vi "Init_queue.vi"(8 "error in (no error)":errorcluster, 9 "response queue":T1, 10 "Name":string, 11 "QueueResponder in":refnum<class "QueueResponder.lvclass">) -> (0 "error out":errorcluster, 3 "QueueResponder out":refnum<class "QueueResponder.lvclass">)   [LabVIEW 2013, in "QueueResponder.lvclass"]
doc: "Initializes the responder. Call before first use"
uses:
  QueueResponder.lvclass
  response queue.ctl
  response.ctl
  driver_status.ctl
  QueueResponder.lvclass/QueueResponder.ctl
  BaseResponder/BaseResponder.lvclass
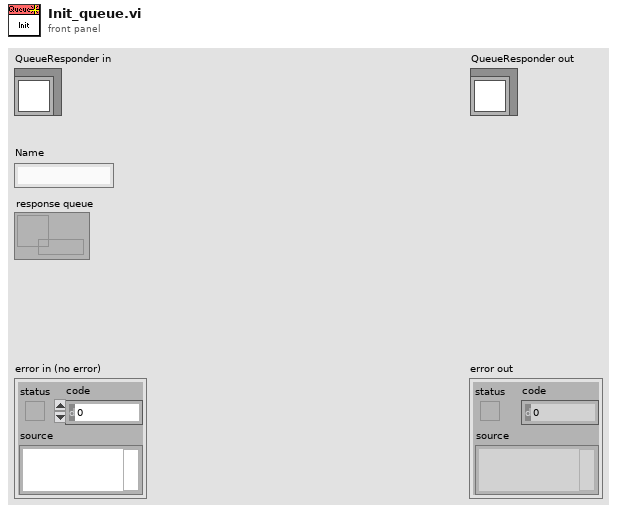
[diagram p1: front panel]
types:
  T1 = typedef "response queue.ctl" = refnum<queue>
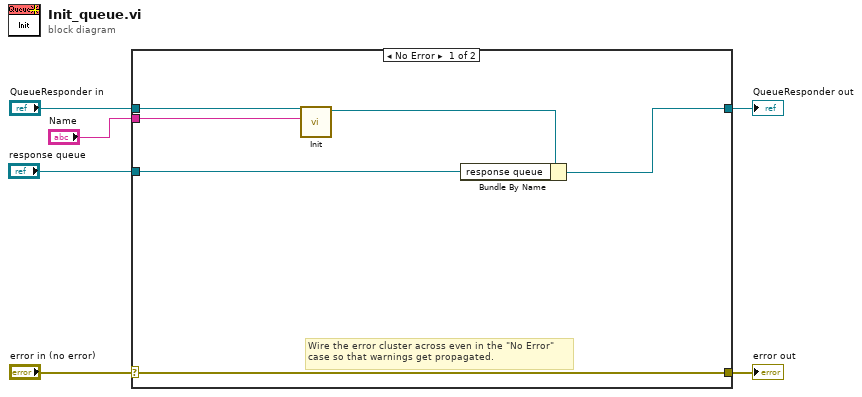
[diagram p0: block diagram]
diagram:
  n1 = case shown="No Error" "error in (no error)" {
    selector: "error in (no error)" -> [w12 w14]
    tunnel: [w12 w14] -> w5
    tunnel: [w11 w13] -> w3
    tunnel: "QueueResponder in" -> [w9 w13]
    tunnel: "response queue" -> [w10 _]
    tunnel: "Name" -> [w7 _]
    frame No Error {
      # "Wire the error cluster across even in the \"No Error\"\ncase so that warnings get propagated."
      n2 = call "Init.vi"("Name"=w7, "BaseResponder in"=w9) -> ("BaseResponder out"=w8:refnum<class "QueueResponder.lvclass">)  [unwired: 8 in, 1 out]
      n3 = Bundle By Name(cluster=w8, "response queue"=w10) -> (w11:refnum<class "QueueResponder.lvclass">)
    }
    frame Error {
    }
  }
  "error out" <- w5
  "QueueResponder out" <- w3
